vi "FPGA_calculate_memadr.vi"(11 "Cluster":cluster{"bus":u8, "channel":u8}) -> (1 "mem adr":u8)   [LabVIEW 2010]
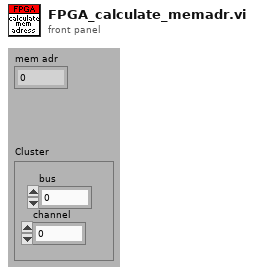
[diagram p1: front panel]
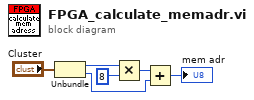
[diagram p0: block diagram]
diagram:
  n1 = Unbundle("Cluster") -> ("bus"=w2:u8, "channel"=w1:u8)
  n2 = Multiply(x=w2, y=u8 8) -> (x*y=w5:u8)
  n3 = Add(x=w5, y=w1) -> (x+y=→"mem adr":u8)
